vi "氨氮质控流程.vi"(7 "队列输入NH3":refnum<queue>, 10 "氨氮":bool, 11 "氨氮量程切换":enum32{"H", "L", "AUTO"}(ring)=enum."AUTO") -> (2 "氨氮中断报警":bool, 3 "布尔":bool)   [LabVIEW 2016, in "质控单元.lvlib"]
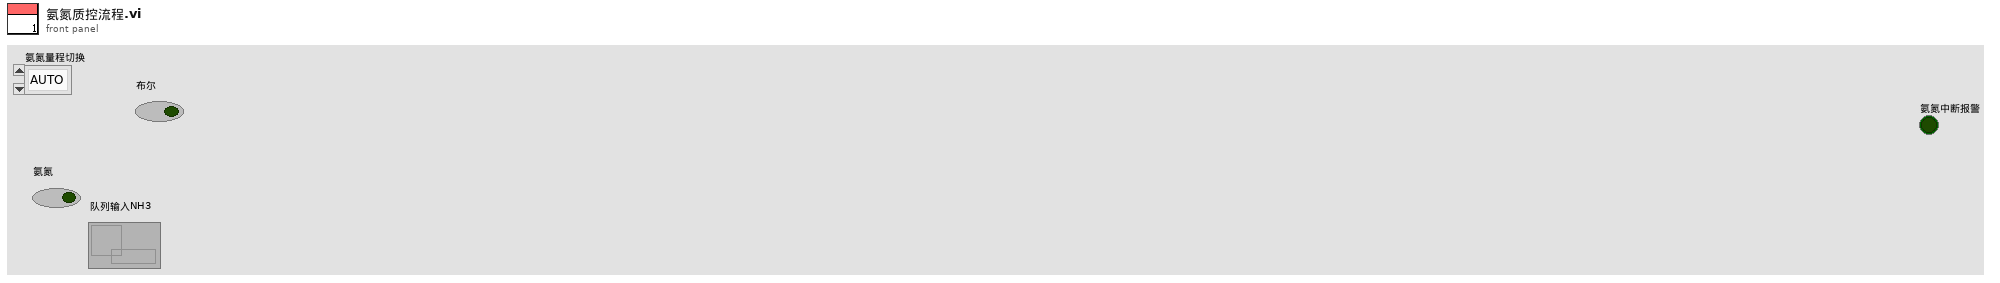
[diagram p1: front panel]
types:
  T1 = enum16{"待机", "启动氨氮水样", "氨氮测量中", "启动氨氮加标", "启动氨氮加标回收", "氨氮加标回收测量中", "启动总氮水样", "总氮测量中", "启动总氮加标", "启动总氮加标回收", "总氮加标回收测量中", "启动总磷水样", "总磷水样测量中", "启动总磷加标", "启动总磷加标回收", "总磷加标回收测量中", "结束"}
  T2 = cluster{"站号":u16, "量程切换":enum32{"H", "L", "AUTO"}, "控制命令":enum16{"启动测量", "标样核查", "零点核查", "跨度核查", "空白测试", "平行样测试", "加标回收", "空白校准", "标样校准", "初始化（清洗）", "停止测试", "仪器重启", "校时", "模式设置", "测量间隔设置"}, "模式设置":enum16{"待机", "连续模式", "周期模式", "定点模式", "受控模式", "手动模式"}, "测量间隔":u16}
  T3 = cluster{"时间标识":timestamp, "设备":string, "日志信息":string}
  T4 = cluster{"系统时间":timestamp, "工作状态":enum16{"空闲", "水样测试", "标样核查", "零点核查", "跨度核查", "空白测试", "平行样测试", "加标回收", "空白校准", "标样校准", "初始化（清洗）"}, "测量模式":enum16{"待机", "连续模式", "周期模式", "定点模式", "受控模式", "手动模式"}, "告警代码":enum16{"无告警", "缺试剂告警", "缺水样告警", "缺蒸馏水告警", "缺标液告警", "仪表漏液告警", "标定异常告警", "超量程告警", "加热异常", "低试剂预警", "超上限告警", "超下限告警", "仪表内部其他异常", "滴定异常告警", "电极异常告警", "量程切换告警", "参数设置告警", "PH电极电位异常", "电导率电极异常", "浊度光度异常", "溶解氧电极异常", "溶解氧光强异常", "温度异常告警", "PH异常告警", "溶解氧异常告警", "电导率异常告警", "浊度异常告警", "叶绿素异常告警", "藻密度异常告警", "蓝绿藻异常告警", "ORP异常告警", "氨氮异常告警", "清洁刷异常告警", "SD卡异常告警", "蓝牙异常告警", "Wifi异常告警", "流程异常告警"}, "故障代码":enum16{"无故障", "电机故障", "温度故障", "通讯故障", "滴定故障"}, "日志代码":u16, "软件版本":u16, "F0":sgl, "F1":sgl, "F2":sgl, "F3":sgl, "T":sgl, "H":sgl, "id":u16, "flowid":u16, "量程":u16, "总磷控温温度1":sgl, "营养盐控温温度2":sgl, "ADC":sgl}
  T5 = enum16{"空闲", "水样测试", "标样核查", "零点核查", "跨度核查", "空白测试", "平行样测试", "加标回收", "空白校准", "标样校准", "初始化（清洗）"}
  T6 = cluster{"因子编码":u32, "单位":u16, "标样参考值":sgl, "水样数据时间":timestamp, "水样实测值":sgl, "水样数据标识":string, "标样数据时间":timestamp, "标样实测值":sgl, "标样数据标识":string, "空白数据时间":timestamp, "空白实测值":sgl, "空白数据标识":string, "零点核查数据时间":timestamp, "零点核查实测值":sgl, "零点核查数据标识":string, "跨度核查数据时间":timestamp, "跨度核查实测值":sgl, "跨度核查数据标识":string, "加标回收数据时间":timestamp, "加标回收实测值":sgl, "加标回收数据标识":string, "平行样数据时间":timestamp, "平行样实测值":sgl, "平行样数据标识":string}
  T7 = cluster{"量程":dbl, "检出限":dbl, "加标前水样浓度":dbl, "加标后水样浓度":dbl, "加标水杯定容体积":dbl, "加标母液浓度":dbl, "加标体积":dbl, "加标回收率":dbl}
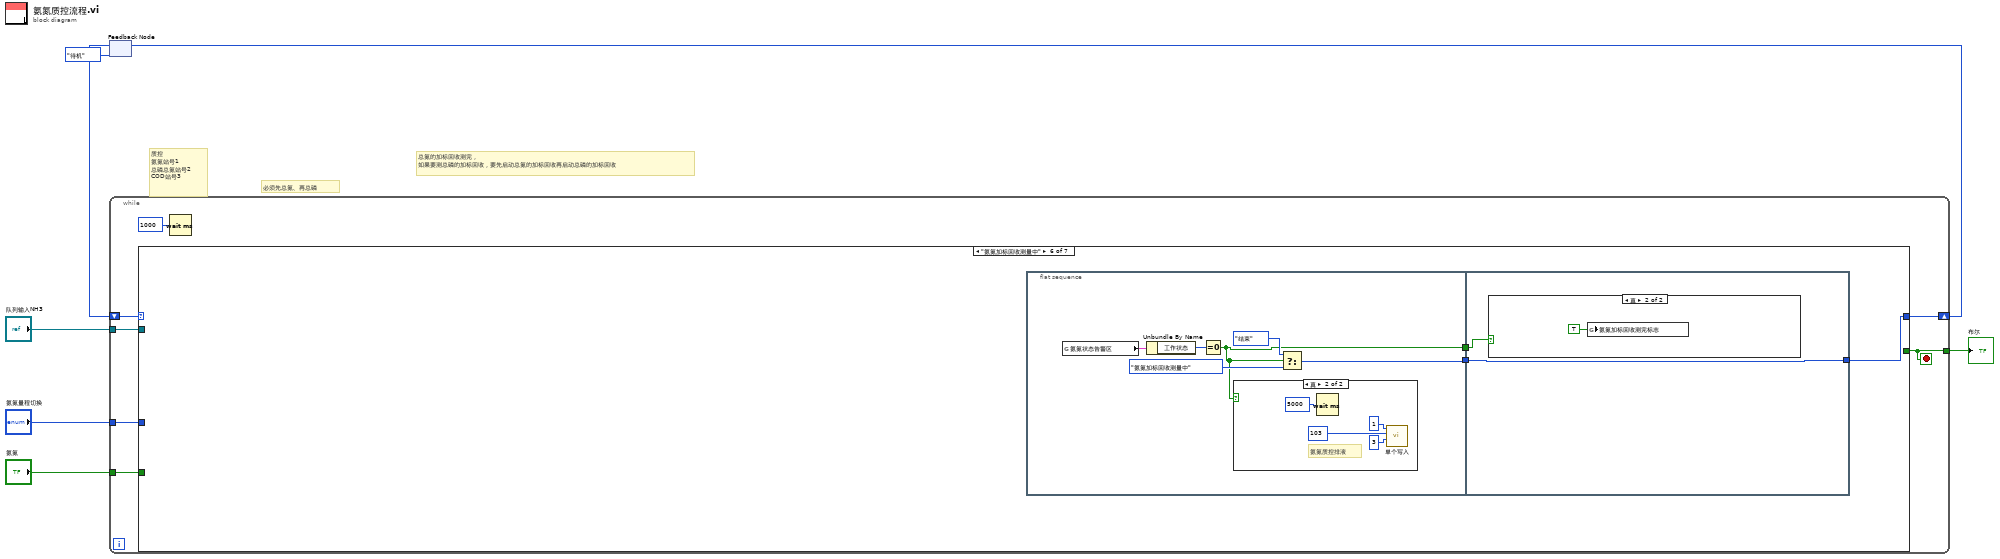
[diagram p0: block diagram]
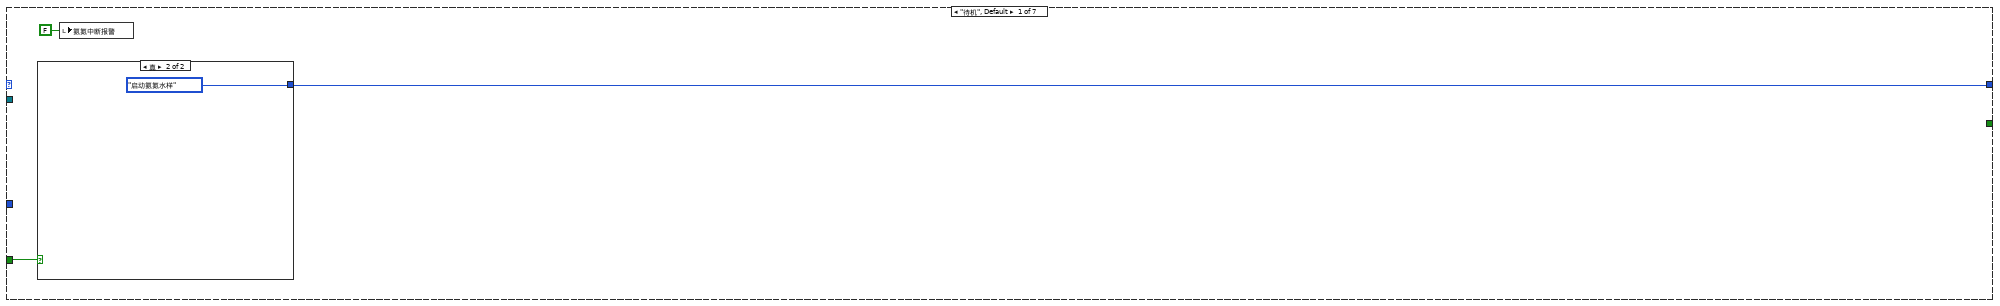
[diagram p2: hidden frame]
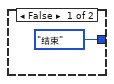
[diagram p3: hidden frame]
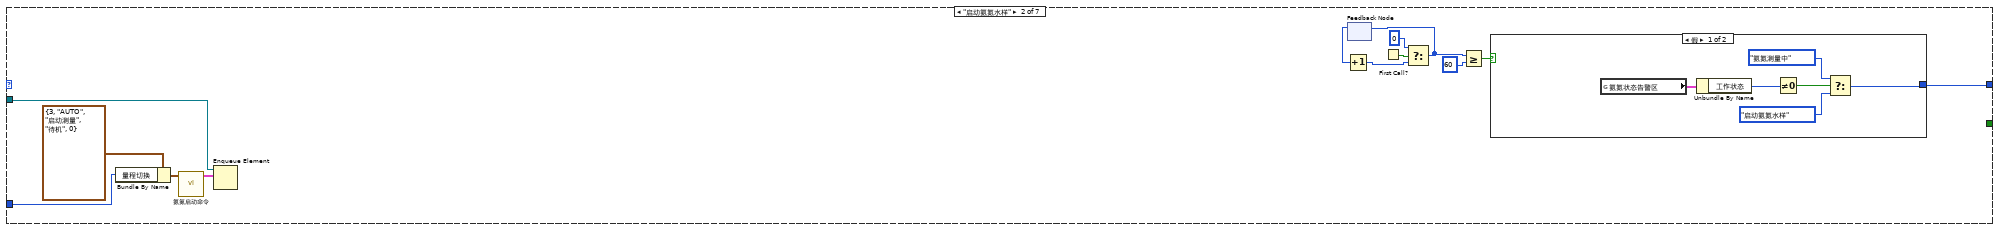
[diagram p4: hidden frame]
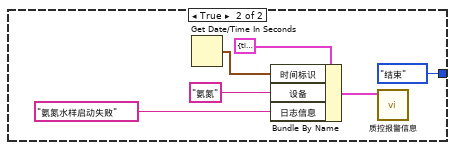
[diagram p5: hidden frame]
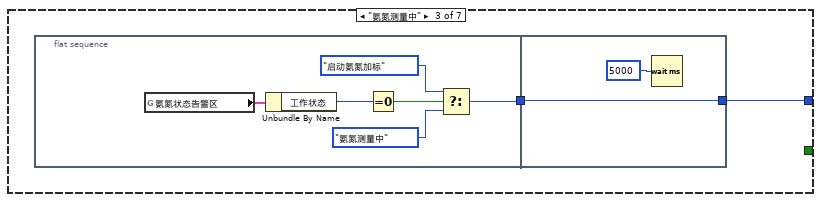
[diagram p6: hidden frame]
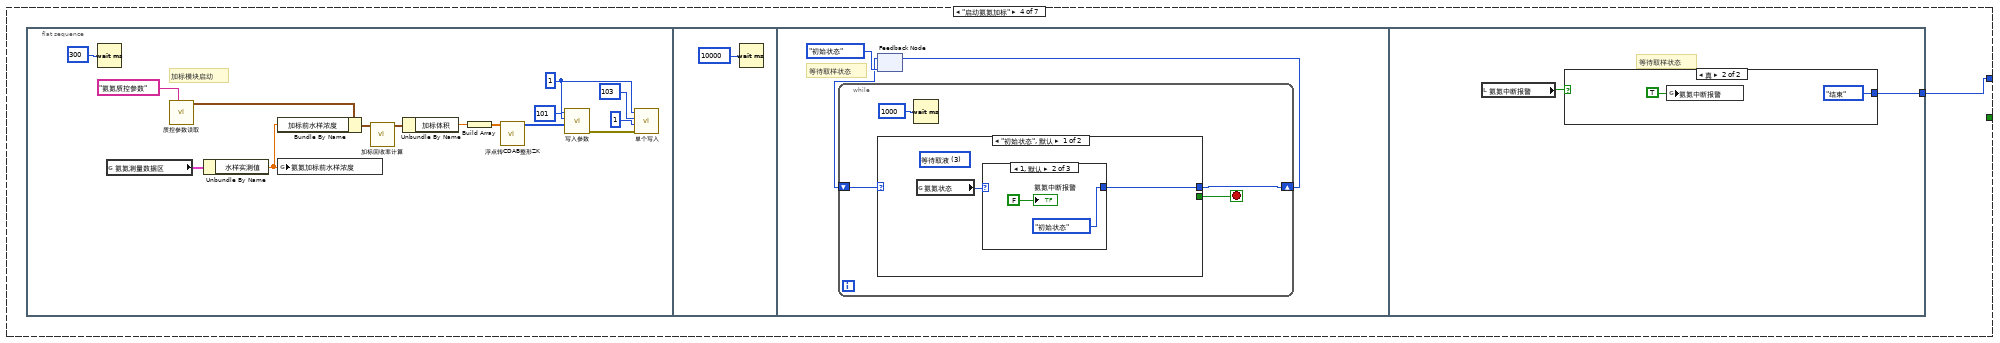
[diagram p7: hidden frame]
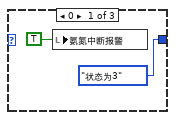
[diagram p8: hidden frame]
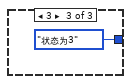
[diagram p9: hidden frame]
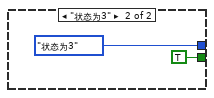
[diagram p10: hidden frame]
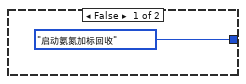
[diagram p11: hidden frame]
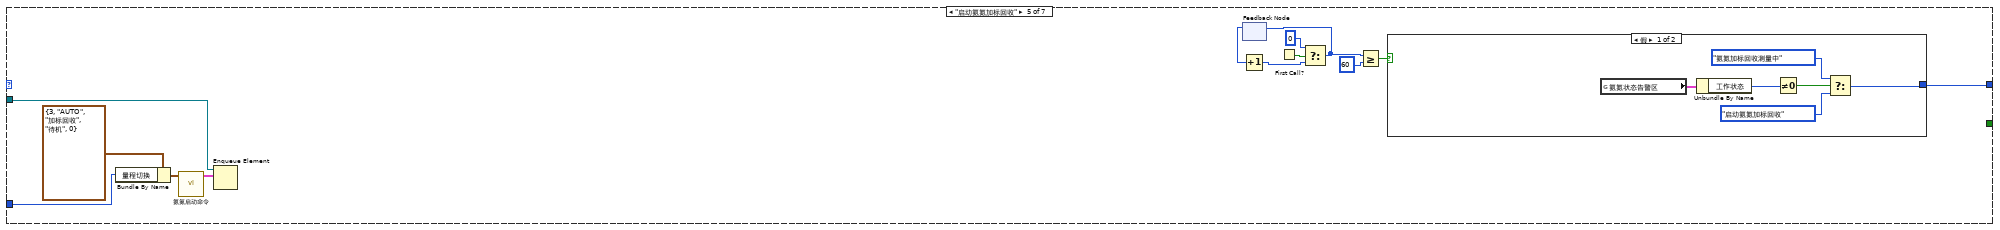
[diagram p12: hidden frame]
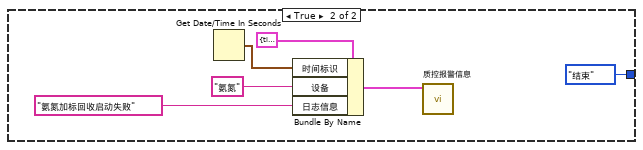
[diagram p13: hidden frame]
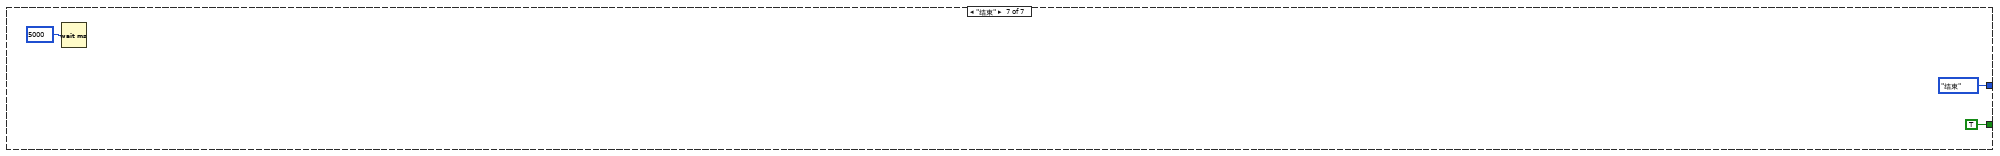
[diagram p16: hidden frame]
diagram:
  # "总氮的加标回收测完，\n如果要测总磷的加标回收，要先启动总氮的加标回收再启动总磷的加标回收"
  # "质控\n氨氮站号1   \n总磷总氮站号2\nCOD站号3"
  # "必须先总氮、再总磷"
  n1 = feedback #1(T1."待机") -> (w1:T1)
  n2 = while {
    tunnel: "队列输入NH3" -> [w12]
    tunnel: "氨氮量程切换" -> [w11]
    tunnel: "氨氮" -> [w14]
    tunnel: [w9] -> w6
    shift-right: [w13] -> w4
    shift-left: w1 -> [w10]
    stop <- w9 stop-if-true
    n3 = case shown="\"氨氮加标回收测量中\"" w10 {
      tunnel: [w17 w32 w46 w55 w98 w119 T1."结束"] -> w13
      tunnel: [_ _ _ _ _ _ TRUE] -> w9
      tunnel: w14 -> [w16 _ _ _ _ _ _]
      tunnel: w12 -> [_ w23 _ _ w96 _ _]
      tunnel: w11 -> [_ w20 _ _ w93 _ _]
      frame "待机", Default {
        n4 = case shown="真" w16 {
          tunnel: [T1."结束" T1."启动氨氮水样"] -> w17
          frame False {
          }
          frame True {
          }
        }
        n5 = local write "氨氮中断报警"(FALSE ("氨氮中断报警")) -> ()
      }
      frame "启动氨氮水样" {
        n6 = Bundle By Name(cluster=T2 {"站号"=3, "量程切换"=enum."AUTO", "控制命令"=enum."启动测量", "模式设置"=enum."待机", "测量间隔"=0} ("参数"), "量程切换"=w20) -> (w21:T2)
        n7 = call "氨氮启动命令.vi"("参数"=w21) -> ("启动命令"=w24:cluster{"命令":string, "data":variant})  [unwired: 10 in]
        n8 = Enqueue Element(queue=w23, element=w24) -> ()  [unwired: 2 in, 3 out]
        n9 = feedback #2() -> (w29:i32)  [unwired: 1 in]
        n10 = Increment(x=w29) -> (x+1=w28:i32)
        n11 = First Call?() -> (First Call?: T/F=w30:bool)
        n12 = Select(t=0, s=w30, f=w28) -> (s? t:f=w27:i32)
        n13 = feedback-in #2(w27) -> ()
        n14 = Greater Or Equal?(x=w27, y=60) -> (x >= y?=w25:bool)
        n15 = case shown="假" w25 {
          tunnel: [w36 T1."结束"] -> w32
          frame False {
            n16 = global read "与氨氮交互全局.vi" "氨氮状态告警区"() -> (w33:T4)
            n17 = Unbundle By Name(w33) -> ("工作状态"=w38:T5)
            n18 = Not Equal To 0?(x=w38) -> (x != 0?=w37:bool)
            n19 = Select(t=T1."氨氮测量中", s=w37, f=T1."启动氨氮水样") -> (s? t:f=w36:T1)
          }
          frame True {
            n20 = Get Date/Time In Seconds() -> (seconds since 1Jan1904=w44:timestamp)
            n21 = Bundle By Name(cluster=T3 {"时间标识"=timestamp(0 s since 1904-01-01), "设备"="", "日志信息"=""} ("data in"), "时间标识"=w44, "设备"="氨氮", "日志信息"="氨氮水样启动失败") -> (w39:T3)
            n22 = call "质控报警信息.vi"("data in"=w39) -> ()  [unwired: 11 in]
          }
        }
      }
      frame "氨氮测量中" {
        n23 = flat-sequence {
          tunnel: [w51] -> w45
          tunnel: [w54] -> w46
          tunnel: w45 -> [w54]
          frame #0 {
            n24 = global read "与氨氮交互全局.vi" "氨氮状态告警区"() -> (w47:T4)
            n25 = Unbundle By Name(w47) -> ("工作状态"=w52:T5)
            n26 = Equal To 0?(x=w52) -> (x = 0?=w50:bool)
            n27 = Select(t=T1."启动氨氮加标", s=w50, f=T1."氨氮测量中") -> (s? t:f=w51:T1)
          }
          frame #1 {
            n28 = Wait (ms)(milliseconds to wait=u32 5000 ("等待时间（毫秒）")) -> ()  [unwired: 1 out]
          }
        }
      }
      frame "启动氨氮加标" {
        n29 = flat-sequence {
          tunnel: [w89] -> w55
          frame #0 {
            w60 = u16 1 ("value")
            # "加标模块启动"
            n30 = Wait (ms)(milliseconds to wait=u32 300 ("等待时间（毫秒）")) -> ()  [unwired: 1 out]
            n31 = global read "与氨氮交互全局.vi" "氨氮测量数据区"() -> (w57:T6)
            n32 = call "质控参数读取.vi"("section"="氨氮质控参数") -> ("参数"=w68:T7)  [unwired: 9 in, 1 out]
            n33 = Unbundle By Name(w57) -> ("水样实测值"=w58:sgl)
            n34 = Bundle By Name(cluster=w68, "加标前水样浓度"=w58) -> (w69:T7)
            n35 = global write "水样浓度全局.vi" "氨氮加标前水样浓度"(w58) -> ()
            n36 = call "加标回收率计算.vi"("参数"=w69) -> ("参数 out"=w67:T7)  [unwired: 10 in]
            n37 = Unbundle By Name(w67) -> ("加标体积"=w59:dbl)
            n38 = Build Array(w59) -> (w66:dbl[])
            n39 = call "浮点转CDAB整形ZK.vi"("浮点数"=w66) -> ("CDAB整形输出"=w61:u16[])  [unwired: 10 in]
            n40 = call "写入参数.vi"("values"=w61, "starting address"=u16 101, "Slave ID"=w60) -> ("error out"=w65:errorcluster)  [unwired: 8 in]
            n41 = call "单个写入.vi"("Error in"=w65, "value"=u16 1, "address"=u16 103, "Slave ID"=w60) -> ()  [unwired: 7 in, 1 out]
          }
          frame #1 {
            n42 = Wait (ms)(milliseconds to wait=u32 10000 ("等待时间（毫秒）")) -> ()  [unwired: 1 out]
          }
          frame #2 {
            # "等待取样状态"
            n43 = feedback #3(enum16{"初始状态", "状态为3"}."初始状态") -> (w73:enum16{"初始状态", "状态为3"})
            n44 = while {
              shift-right: [w77] -> w72
              shift-left: w73 -> [w78]
              stop <- w76 stop-if-true
              n45 = case shown="\"初始状态\", 默认" w78 {
                tunnel: [w80 enum16{"初始状态", "状态为3"}."状态为3"] -> w77
                tunnel: [_ TRUE] -> w76
                frame "初始状态", Default {
                  (unwired) u16 3 items=["待机", "润洗", "进样", "等待取液", "排液"] ("氨氮状态")
                  n46 = global read "加标回收状态全局变量.vi" "氨氮状态"() -> (w79:u16)
                  n47 = case shown="1, 默认" w79 {
                    tunnel: [enum16{"初始状态", "状态为3"}."状态为3" enum16{"初始状态", "状态为3"}."初始状态" enum16{"初始状态", "状态为3"}."状态为3"] -> w80
                    frame 0 {
                      n48 = local write "氨氮中断报警"(TRUE ("氨氮中断报警")) -> ()
                    }
                    frame 1, Default {
                      "氨氮中断报警" <- FALSE ("总氮中断报警")
                    }
                    frame 3 {
                    }
                  }
                }
                frame "状态为3" {
                }
              }
              n49 = Wait (ms)(milliseconds to wait=u32 1000 ("等待时间（毫秒）")) -> ()  [unwired: 1 out]
            }
            n50 = feedback-in #3(w72) -> ()
          }
          frame #3 {
            # "等待取样状态"
            n51 = local read "氨氮中断报警"() -> (w88:bool)
            n52 = case shown="真" w88 {
              tunnel: [T1."启动氨氮加标回收" T1."结束"] -> w89
              frame False {
              }
              frame True {
                n53 = global write "质控中断报警全局.vi" "氨氮中断报警"(TRUE ("氨氮中断报警")) -> ()
              }
            }
          }
        }
      }
      frame "启动氨氮加标回收" {
        n54 = Bundle By Name(cluster=T2 {"站号"=3, "量程切换"=enum."AUTO", "控制命令"=enum."加标回收", "模式设置"=enum."待机", "测量间隔"=0} ("参数"), "量程切换"=w93) -> (w94:T2)
        n55 = call "氨氮启动命令.vi"("参数"=w94) -> ("启动命令"=w97:cluster{"命令":string, "data":variant})  [unwired: 10 in]
        n56 = Enqueue Element(queue=w96, element=w97) -> ()  [unwired: 2 in, 3 out]
        n57 = feedback #4() -> (w103:i32)  [unwired: 1 in]
        n58 = Increment(x=w103) -> (x+1=w102:i32)
        n59 = First Call?() -> (First Call?: T/F=w104:bool)
        n60 = Select(t=0, s=w104, f=w102) -> (s? t:f=w101:i32)
        n61 = feedback-in #4(w101) -> ()
        n62 = Greater Or Equal?(x=w101, y=60) -> (x >= y?=w99:bool)
        n63 = case shown="假" w99 {
          tunnel: [w109 T1."结束"] -> w98
          frame False {
            n64 = global read "与氨氮交互全局.vi" "氨氮状态告警区"() -> (w106:T4)
            n65 = Unbundle By Name(w106) -> ("工作状态"=w111:T5)
            n66 = Not Equal To 0?(x=w111) -> (x != 0?=w110:bool)
            n67 = Select(t=T1."氨氮加标回收测量中", s=w110, f=T1."启动氨氮加标回收") -> (s? t:f=w109:T1)
          }
          frame True {
            n68 = Get Date/Time In Seconds() -> (seconds since 1Jan1904=w117:timestamp)
            n69 = Bundle By Name(cluster=T3 {"时间标识"=timestamp(0 s since 1904-01-01), "设备"="", "日志信息"=""} ("data in"), "时间标识"=w117, "设备"="氨氮", "日志信息"="氨氮加标回收启动失败") -> (w112:T3)
            n70 = call "质控报警信息.vi"("data in"=w112) -> ()  [unwired: 11 in]
          }
        }
      }
      frame "氨氮加标回收测量中" {
        n71 = flat-sequence {
          tunnel: [w125] -> w120
          tunnel: [w121] -> w118
          tunnel: [w132] -> w119
          tunnel: w120 -> [w132]
          tunnel: w118 -> [w131]
          frame #0 {
            n72 = global read "与氨氮交互全局.vi" "氨氮状态告警区"() -> (w122:T4)
            n73 = Unbundle By Name(w122) -> ("工作状态"=w126:T5)
            n74 = Equal To 0?(x=w126) -> (x = 0?=w121:bool)
            n75 = case shown="真" w121 {
              frame False {
              }
              frame True {
                # "氨氮质控排液"
                n76 = Wait (ms)(milliseconds to wait=u32 5000 ("等待时间（毫秒）")) -> ()  [unwired: 1 out]
                n77 = call "单个写入.vi"("value"=u16 3, "address"=u16 103, "Slave ID"=u8 1) -> ()  [unwired: 8 in, 1 out]
              }
            }
            n78 = Select(t=T1."结束", s=w121, f=T1."氨氮加标回收测量中") -> (s? t:f=w125:T1)
          }
          frame #1 {
            n79 = case shown="真" w131 {
              frame False {
              }
              frame True {
                n80 = global write "质控测完标志全局 1.vi" "氨氮加标回收测完标志"(TRUE) -> ()
              }
            }
          }
        }
      }
      frame "结束" {
        n81 = Wait (ms)(milliseconds to wait=u32 5000 ("等待时间（毫秒）")) -> ()  [unwired: 1 out]
      }
    }
    n82 = Wait (ms)(milliseconds to wait=u32 1000 ("等待时间（毫秒）")) -> ()  [unwired: 1 out]
  }
  "布尔" <- w6
  n83 = feedback-in #1(w4) -> ()
